vi "Configure ECU PWM Shifter with Null.vi"(8 "error in (no error)":errorcluster, 9 "NIVS.System Definition Root":refnum<k24>, 10 "VI Reference":refnum<vi>, 11 "FNR Data in":T1) -> (0 "error out":errorcluster, 3 "FNR Data Out":T1)   [LabVIEW 2013]
doc: "Use this template to create a dialog box with event handling."
uses:
  NationalInstruments.VeriStand.SystemStorageUI
  NationalInstruments.VeriStand.SystemStorage
  Support/FNR Object Parameters.ctl
  Support/PWM Object Parameters.ctl
  <vilib>/NI Veristand/UI Controls/Single Node Browser/NI_VS UI Single Node Browser.lvlib
panel:
  in  "Null PWM":dbl format="%#.6f"
  in  "Make Current Values Default":bool
  in  "Reverse PWM":dbl=10.0 format="%#.6f"
  in  "Neutral PWM":dbl=25.0 format="%#.6f"
  in  "Forward PWM":dbl=100.0 format="%#.6f"
  in  "BG color":u32(colorbox)=16777228
  in  "Control Color":u32(colorbox)=16761088
  in  "Control Label":string
  in  "OK":bool
  in  "Cancel":bool
  in  "Selected Channel":refnum<k24>(container)
  # "Output Values"
  # "F"
  # "N"
  # "R"
  # "NULL"
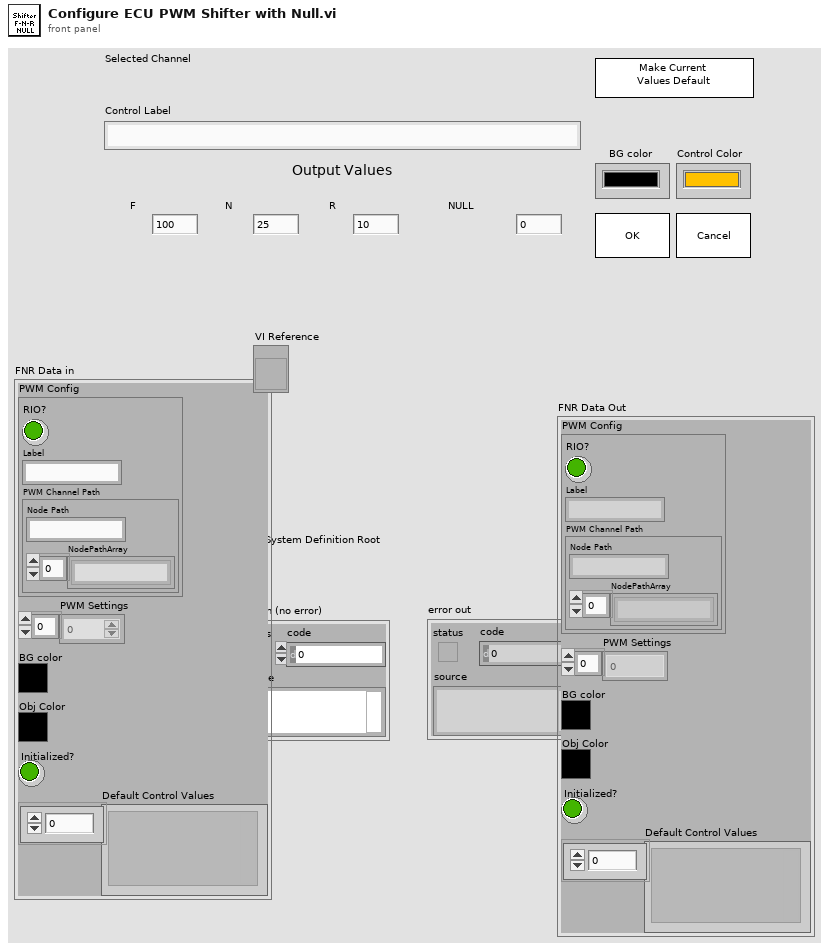
[diagram p1: front panel]
types:
  T1 = typedef "FNR Object Parameters.ctl" = cluster{"PWM Config":T2, "PWM Settings":dbl[], "BG color":u32, "Obj Color":u32, "Initialized?":bool, "Default Control Values":variant[]}
  T2 = typedef "PWM Object Parameters.ctl" = cluster{"RIO?":bool, "Label":string, "PWM Channel Path":cluster{"NodePathArray":string[], "Node Path":string}}
  T3 = typedef "NI_VS UI Single Node Browser.lvlib/Callback Type.ctl" = cluster{"Net Callbacks":refnum<k27>[], "Event":refnum<user-event>}
  T4 = typedef "NI_VS UI Single Node Browser.lvlib/Node Ref.ctl" = refnum<k24>
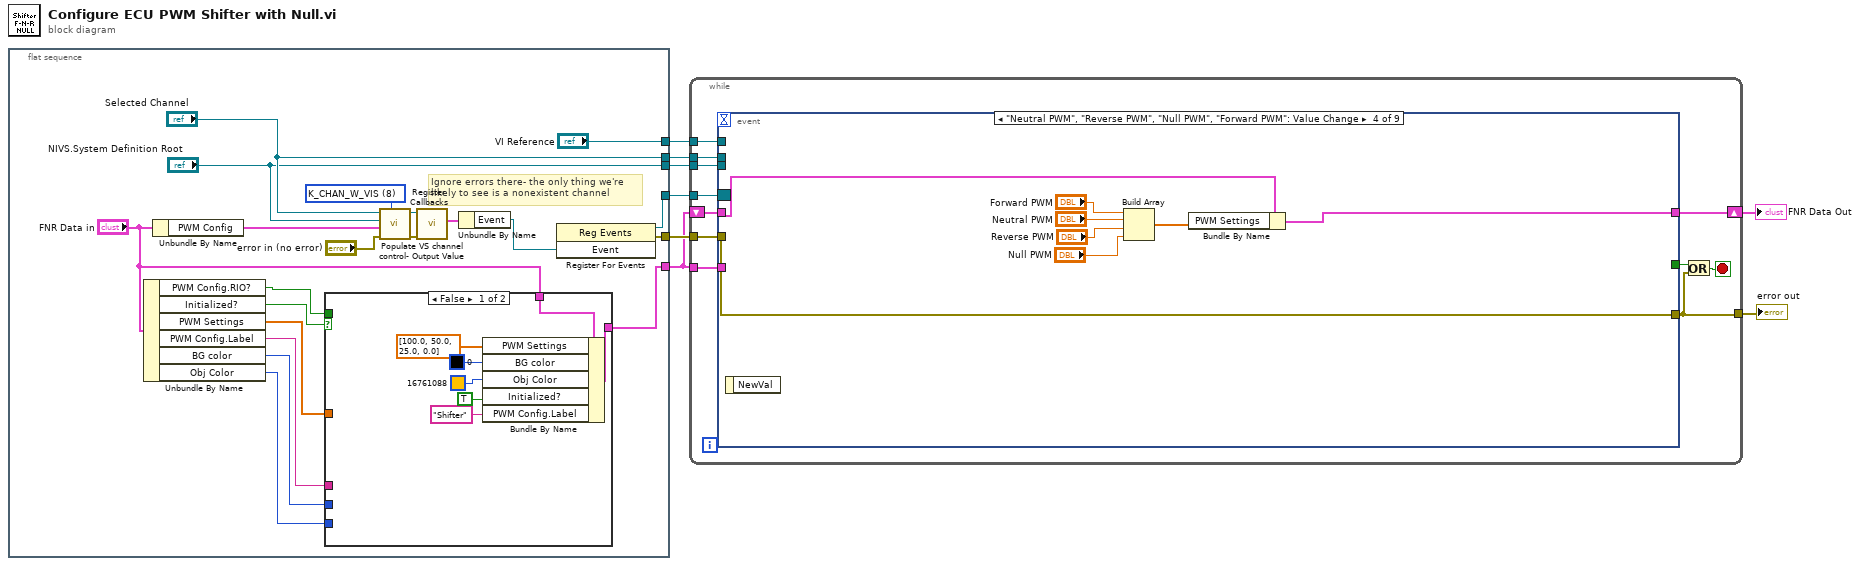
[diagram p0: block diagram]
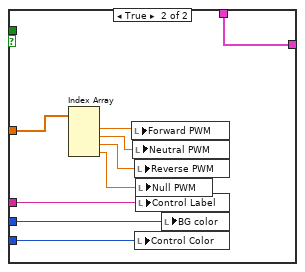
[diagram p2: hidden frame]
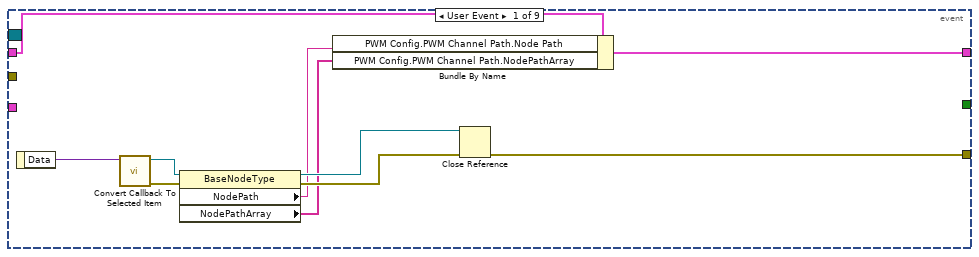
[diagram p3: hidden frame]
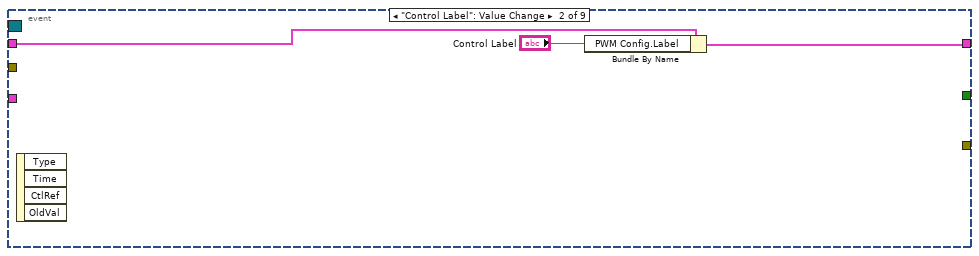
[diagram p4: hidden frame]
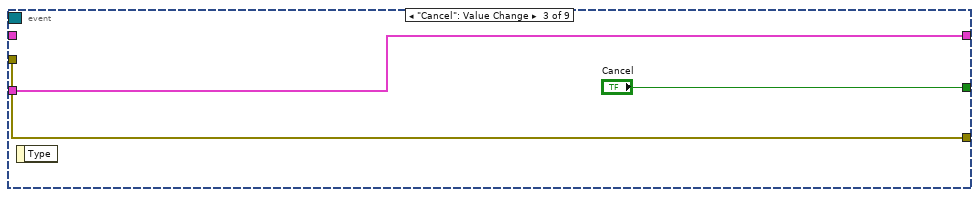
[diagram p5: hidden frame]
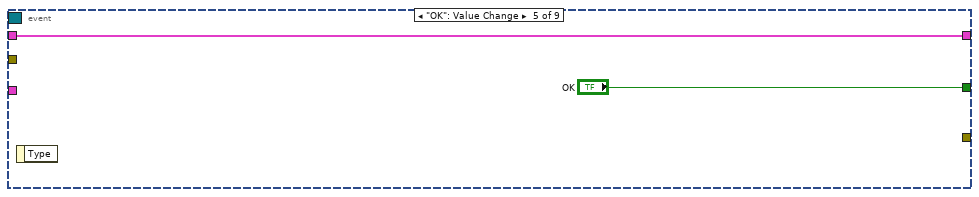
[diagram p6: hidden frame]
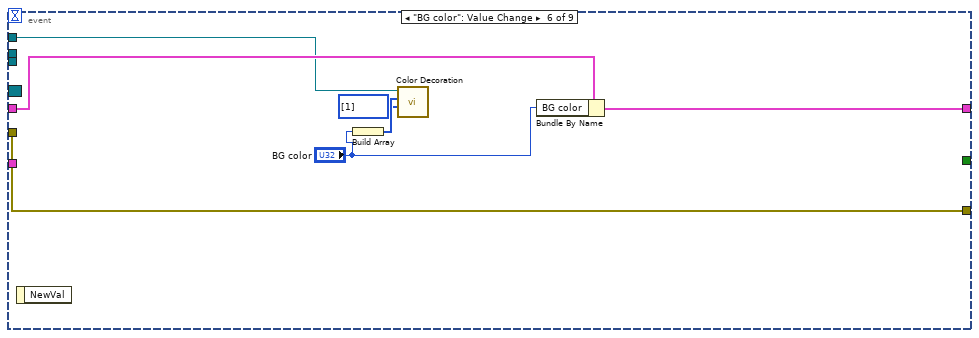
[diagram p7: hidden frame]
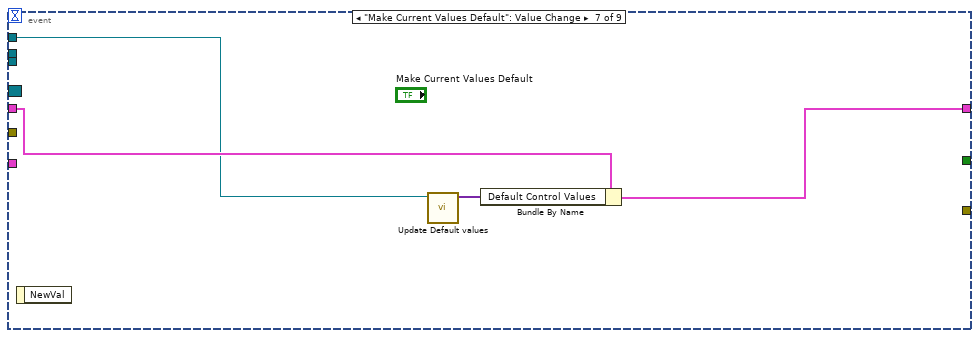
[diagram p8: hidden frame]
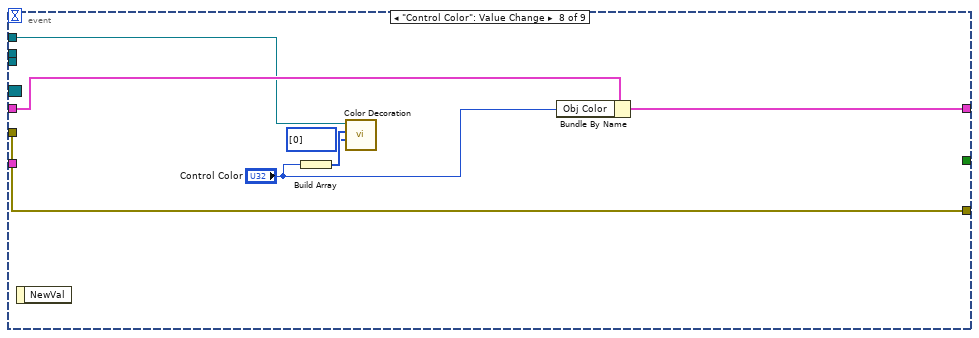
[diagram p9: hidden frame]
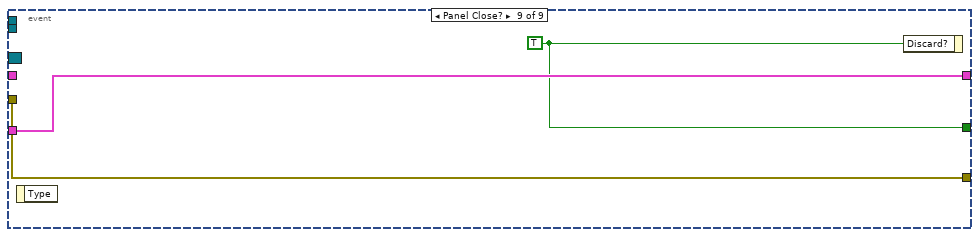
[diagram p10: hidden frame]
diagram:
  n1 = flat-sequence {
    tunnel: ["Selected Channel"] -> w7
    tunnel: ["NIVS.System Definition Root"] -> w6
    tunnel: [w12] -> w5
    tunnel: [w18] -> w3
    tunnel: ["VI Reference"] -> w2
    tunnel: [w11] -> w1
    frame #0 {
      w27 = u8 8 items=["K_CHAN_R", "K_CHAN_W", "K_CHAN_RW", "K_CHAN_VOLT", "K_CHAN_FAULT", "K_ALL", "K_CUSTOM", "K_CHAN_R_VIS", "K_CHAN_W_VIS", "K_CHAN_RW_VIS", "K_CHAN_VOLT_VIS", "K_CHAN_FAULT_VIS"] ("DisplayFilter")
      # "Ignore errors there- the only thing we're\nlikely to see is a nonexistent channel"
      n2 = Unbundle By Name("FNR Data in") -> ("PWM Config.RIO?"=w10:bool, "Initialized?"=w20:bool, "PWM Settings"=w24:dbl[], "PWM Config.Label"=w23:string, "BG color"=w22:u32, "Obj Color"=w21:u32)
      n3 = Unbundle By Name("FNR Data in") -> ("PWM Config"=w26:T2)
      n4 = case shown="False" w20 {
        tunnel: w24 -> [_ w41]
        tunnel: w23 -> [_ w40]
        tunnel: w22 -> [_ w39]
        tunnel: w21 -> [_ w38]
        tunnel: "FNR Data in" -> [w35 w37]
        tunnel: [w34 w37] -> w18
        tunnel: w10 -> [_ _]
        frame False {
          n5 = Bundle By Name(cluster=w35, "PWM Settings"=dbl[] [100.0, 50.0, 25.0, 0.0] ("RIO PWM Settings"), "BG color"=u32 0, "Obj Color"=u32 16761088, "Initialized?"=TRUE ("New?"), "PWM Config.Label"="Shifter" ("Label")) -> (w34:T1)
        }
        frame True {
          n6 = Index Array(array=w41) -> (element #1=w44:dbl, element #2=w43:dbl, element #3=w42:dbl, element #4=w36:dbl)  [unwired: 4 in]
          n7 = local write "Forward PWM"(w44) -> ()
          n8 = local write "Neutral PWM"(w43) -> ()
          n9 = local write "Reverse PWM"(w42) -> ()
          n10 = local write "Control Color"(w38) -> ()
          n11 = local write "Null PWM"(w36) -> ()
          n12 = local write "Control Label"(w40) -> ()
          n13 = local write "BG color"(w39) -> ()
        }
      }
      n14 = call "Populate VS channel control- Output Value.vi"("DisplayFilter"=w27, "error in (no error)"="error in (no error)", "Data cluster in"=w26, "NIVS.System Definition Root"="NIVS.System Definition Root", ".NET Refnum in"="Selected Channel") -> ("error out"=w13:errorcluster, ".NET Refnum out"=w14:refnum<k24>)  [unwired: 5 in]
      n15 = call <vilib>:"Register Callbacks.vi"("error in (no error)"=w13, "Single Node Browser"=w14) -> ("Callbacks"=w16:T3)  [unwired: 7 in, 2 out]
      n16 = Unbundle By Name(w16) -> ("Event"=w15:refnum<user-event>)
      n17 = register-events(w15) -> (reference out=w11:refnum<event-registration>, error out=w12:errorcluster)  [unwired: 2 in]
    }
  }
  n18 = while {
    tunnel: [w45] -> w8
    shift-right: [w52] -> w4
    shift-left: w3 -> [w54]
    tunnel: w3 -> [w53]
    tunnel: w7 -> [w50]
    tunnel: w6 -> [w49]
    tunnel: w5 -> [w48]
    tunnel: w2 -> [w47]
    tunnel: w1 -> [w46]
    stop <- w51 stop-if-true
    n19 = event shown="[3] \"Neutral PWM\", \"Reverse PWM\", \"Null PWM\", \"Forward PWM\": Value Change" {
      selector: w46 -> [_ _ _ _ _ _ _ _ _]
      dyn-events: _ -> [_ _ _ _ _ _ _ _ _]
      timeout: _ -> [_ _ _ _ _ _ _ _ _]
      tunnel: [_ _ "Cancel" _ "OK" _ _ _ w101] -> w55
      tunnel: [w57 _ w69 w79 _ w86 _ w97 w100] -> w45
      tunnel: w54 -> [w58 w67 _ w78 w80 w87 w91 w98 _]
      tunnel: w53 -> [_ _ w70 _ _ _ _ _ w102]
      tunnel: [w56 w68 w70 w77 w80 w88 w90 w99 w102] -> w52
      tunnel: w50 -> [_ _ _ _ _ _ _ _ _]
      tunnel: w49 -> [_ _ _ _ _ _ _ _ _]
      tunnel: w48 -> [_ _ w69 w79 _ w86 _ w97 w100]
      tunnel: w47 -> [_ _ _ _ _ w82 w89 w93 _]
      event User Event {
        n20 = event-data() -> ("Data"=w59:variant)  [unwired: 1 in]
        n21 = call <vilib>:"Convert Callback To Selected Item.vi"("Data"=w59) -> ("error out"=w62:errorcluster, "Selected Item"=w65:T4)  [unwired: 9 in]
        n22 = property class="BaseNodeType"(reference=w65, error in=w62) -> (reference out=w64:T4, error out=w63:errorcluster, "NodePath"=w61:string, "NodePathArray"=w60:string[])
        n23 = Bundle By Name(cluster=w58, "PWM Config.PWM Channel Path.Node Path"=w61, "PWM Config.PWM Channel Path.NodePathArray"=w60) -> (w56:T1)
        n24 = Close Reference(reference=w64, error in (no error)=w63) -> (error out=w57:errorcluster)
      }
      event "Control Label": Value Change {
        n25 = event-data() -> ()  [unwired: 1 in, 4 out]
        n26 = Bundle By Name(cluster=w67, "PWM Config.Label"="Control Label") -> (w68:T1)
      }
      event "Cancel": Value Change {
        n27 = event-data() -> ()  [unwired: 1 in, 1 out]
      }
      event "Neutral PWM", "Reverse PWM", "Null PWM", "Forward PWM": Value Change {
        n28 = event-data() -> ()  [unwired: 1 in, 1 out]
        n29 = Build Array("Forward PWM", "Neutral PWM", "Reverse PWM", "Null PWM") -> (w73:dbl[])
        n30 = Bundle By Name(cluster=w78, "PWM Settings"=w73) -> (w77:T1)
      }
      event "OK": Value Change {
        n31 = event-data() -> ()  [unwired: 1 in, 1 out]
      }
      event "BG color": Value Change {
        n32 = event-data() -> ()  [unwired: 1 in, 1 out]
        n33 = Build Array("BG color") -> (w85:u32[])
        n34 = call "Color Decoration.vi"("VI reference"=w82, "Color Array"=w85, "Index Array"=u32[] [1]) -> ()  [unwired: 7 in, 1 out]
        n35 = Bundle By Name(cluster=w87, "BG color"="BG color") -> (w88:T1)
      }
      event "Make Current Values Default": Value Change {
        n36 = event-data() -> ()  [unwired: 1 in, 1 out]
        n37 = call "Update Default values.vi"("VI in"=w89) -> ("Default Values out"=w92:variant[])  [unwired: 10 in]
        n38 = Bundle By Name(cluster=w91, "Default Control Values"=w92) -> (w90:T1)
      }
      event "Control Color": Value Change {
        n39 = event-data() -> ()  [unwired: 1 in, 1 out]
        n40 = Build Array("Control Color") -> (w96:u32[])
        n41 = call "Color Decoration.vi"("VI reference"=w93, "Color Array"=w96, "Index Array"=u32[] [0]) -> ()  [unwired: 7 in, 1 out]
        n42 = Bundle By Name(cluster=w98, "Obj Color"="Control Color") -> (w99:T1)
      }
      event Panel Close? {
        w101 = TRUE ("Cancel")
        n43 = event-data() -> ()  [unwired: 1 in, 1 out]
        n44 = event-data("Discard?"=w101) -> ()  [unwired: 1 in, 1 out]
      }
    }
    n45 = Or(x=w55, y=w45) -> (x .or. y?=w51:bool)
  }
  "error out" <- w8
  "FNR Data Out" <- w4
